vi "Name.vi"(8 "error in (no error)":errorcluster, 11 "FormField in":refnum<class "FormField.lvclass">) -> (0 "error out":errorcluster, 2 "Name":string, 3 "FormField out":refnum<class "FormField.lvclass">)   [LabVIEW 2020, in "HTTP Utils.lvlib" / "FormField.lvclass"]
uses:
  FormField.lvclass
  FormField.lvclass/FormField.ctl
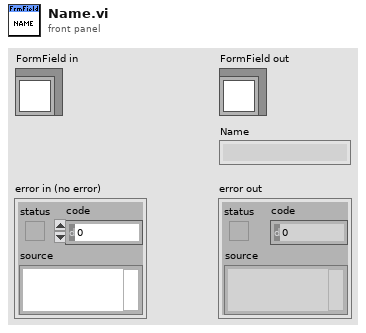
[diagram p1: front panel]
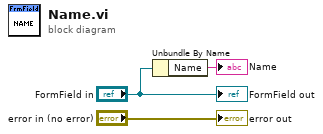
[diagram p0: block diagram]
diagram:
  n1 = Unbundle By Name("FormField in") -> ("Name"=→"Name":string)
  "error out" <- "error in (no error)"
  "FormField out" <- "FormField in"
